vi "local.Set NVMEM Bytes.vi"(0 "SLSC Local in":refnum<class "SLSC Interface.lvclass">, 5 "NVMEM area":refnum<k21>="$DefaultNVMEMAreas", 7 "data address":u32 format="%.0x", 9 "data":u8[](array[numeric]) format="%.0x", 11 "error in (no error)":errorcluster) -> (4 "SLSC Local out":refnum<class "SLSC Interface.lvclass">, 6 "NVMEM area out":refnum<k21>, 8 "next data address":u32 format="%.0x", 15 "error out":errorcluster)   [LabVIEW 2016, in "SLSC Interfaces.lvlib" / "SLSC Interface.lvclass"]
uses:
  SLSC Interface Class/SLSC Interface.lvclass
  <vilib>/SLSC/SLSC.lvlib
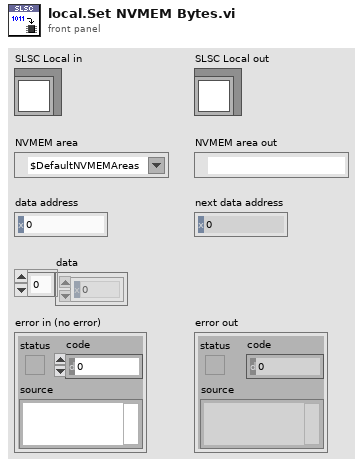
[diagram p1: front panel]
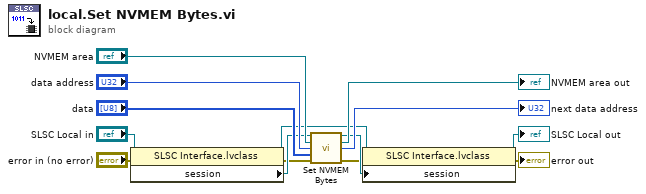
[diagram p0: block diagram]
diagram:
  n1 = property class="SLSC Interface.lvclass"(reference="SLSC Local in", error in="error in (no error)") -> (reference out=w8:refnum<class "SLSC Interface.lvclass">, error out=w3:errorcluster, "session"=w6:refnum<k21>)
  n2 = call <vilib>:"Set NVMEM Bytes.vi"("session in"=w6, "NVMEM area"="NVMEM area", "data address"="data address", "data"="data", "error in (no error)"=w3) -> ("session out"=w5:refnum<k21>, "NVMEM area out"=→"NVMEM area out":refnum<k21>, "next data address"=→"next data address":u32, "error out"=w2:errorcluster)  [unwired: 7 in]
  n3 = property class="SLSC Interface.lvclass"(reference=w8, error in=w2, "session"=w5) -> (reference out=→"SLSC Local out":refnum<class "SLSC Interface.lvclass">, error out=→"error out":errorcluster)
